vi "Configure RMS Current Limits.vi"(0 "VISA resource name":refnum<visa-resource-name>, 5 "Current Low Limit (0 A)":dbl min=0.0 max=36.8 format="%.3f", 7 "Current High Limit (0 A)":dbl min=0.0 max=36.8 format="%.3f", 11 "error in (no error)":errorcluster) -> (4 "VISA resource name out":refnum<visa-resource-name>, 15 "error out":errorcluster)   [LabVIEW 2014, in "eec 6700.lvlib"]
doc: "Configure the current (rms) limits in the active step of the power source instrument.\n\n<B>Range</B> : 0.000~33.60 A\n\n Model | Voltage Range | RMS Current\n------------------------------------------------\n 6705 | (0-150 V) - Auto | 0.00 - 4.20 A\n 6705 | (0-300 V) - High | 0.00 - 2.10 A\n---------------------------------------------\n 6710 | (0-150 V) - Auto | 0.00 - 8.40 A\n 6710 | (0-300 V) - High | 0.00 - 4.20 A\n--------------------------------------\n 6720 | (0-150 V) - Auto | 0.00 - 16.80 A\n 6720 | (0-300 V) - High | 0.00 - 8.40 A\n--------------------------------------\n 6730 | (0-150 V) - Auto | 0.00 - 25.20 A\n 6730 | (0-300 V) - High | 0.00 - 12.60 A\n--------------------------------------\n 6740 | (0-150 V) - Auto | 0.00 - 33.60 A\n 6740 | (0-300 V) - High | 0.00 - 16.80 A\n\nThe current Limit setting configures a current threshold level. A test failure will occur when the high limit is reached or the low limit is not reached.\n\nNote : This VI can be used only for Program Mode.\nRun \"Configure Program Mode.vi\" to make sure the instrument is in <B>Program Mode</B> before using this VI"
uses:
  <instrlib>/eec 6700/eec 6700.lvlib
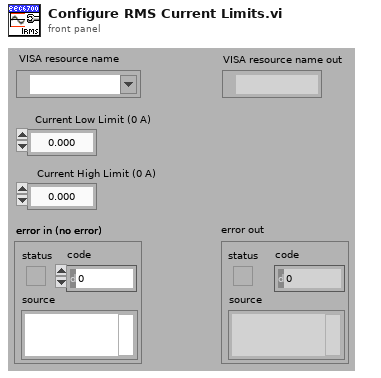
[diagram p1: front panel]
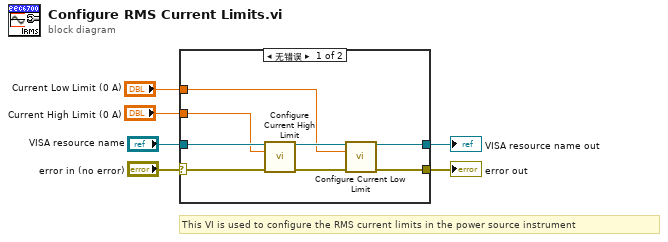
[diagram p0: block diagram]
diagram:
  # "This VI is used to configure the RMS current limits in the power source instrument"
  n1 = case shown="无错误" "error in (no error)" {
    selector: "error in (no error)" -> [w11 w16]
    tunnel: [w8 w16] -> w6
    tunnel: [w7 w15] -> w5
    tunnel: "VISA resource name" -> [w12 w15]
    tunnel: "Current High Limit (0 A)" -> [w10 _]
    tunnel: "Current Low Limit (0 A)" -> [w9 _]
    frame No Error {
      n2 = call <instrlib>:"Configure Current High Limit.vi"("VISA resource name"=w12, "Current High Limit (0 A)"=w10, "error in (no error)"=w11) -> ("VISA resource name out"=w13:refnum<visa-resource-name>, "error out"=w14:errorcluster)  [unwired: 11 in]
      n3 = call <instrlib>:"Configure Current Low Limit.vi"("VISA resource name"=w13, "Current Low Limit (0 A)"=w9, "error in (no error)"=w14) -> ("VISA resource name out"=w7:refnum<visa-resource-name>, "error out"=w8:errorcluster)  [unwired: 11 in]
    }
    frame Error {
    }
  }
  "error out" <- w6
  "VISA resource name out" <- w5
